vi "Agitator Tags.vi"(11 "AM Module Configs":T1[](array[typedef])) -> (1 "AG Tags":T4, 2 "AM Module Tags Array":T4[](array[typedef]), 3 "All Boolean Tags":string[](array[string]), 4 "All  Numeric Tags":string[](array[string]))   [LabVIEW 2018]
uses:
  Agitator Class/Agitator Module Tag Names.ctl
  Agitator Module Folder/Feed Module/Controls/Agitator Module Config Cluster.ctl
  <vilib>/Utility/miscctls.llb/LVPoint32TypeDef.ctl
  Agitator Module Folder/Feed Module/Controls/Agitator Module Settings Cluster.ctl
  Agitator Module Folder/Agitator Module.lvlib
panel:
  # "Agitator Settings"
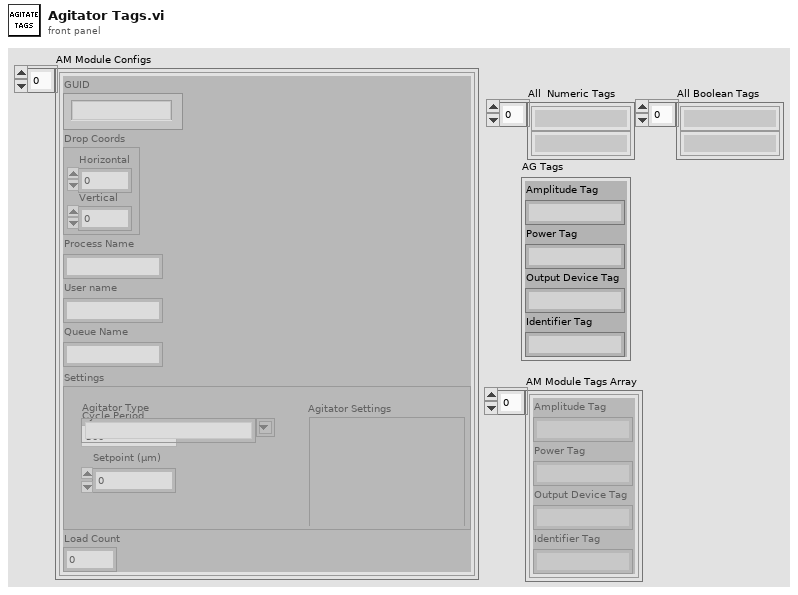
[diagram p1: front panel]
types:
  T1 = typedef "Agitator Module.lvlib/Agitator Module Config Cluster.ctl" = cluster{"GUID":string, "Drop Coords":T2, "Process Name":string, "User name":string, "Queue Name":string, "Settings":T3, "Load Count":i32}
  T2 = typedef "LVPoint32TypeDef.ctl" = cluster{"Horizontal":i32, "Vertical":i32}
  T3 = typedef "Agitator Module.lvlib/Agitator Module Settings Cluster.ctl" = cluster{"Cycle Period":dbl, "Agitator Type":string, "Setpoint (µm)":dbl}
  T4 = typedef "Agitator Module.lvlib/Agitator Module Tag Names.ctl" = cluster{"Amplitude Tag":string, "Power Tag":string, "Output Device Tag":string, "Identifier Tag":string}
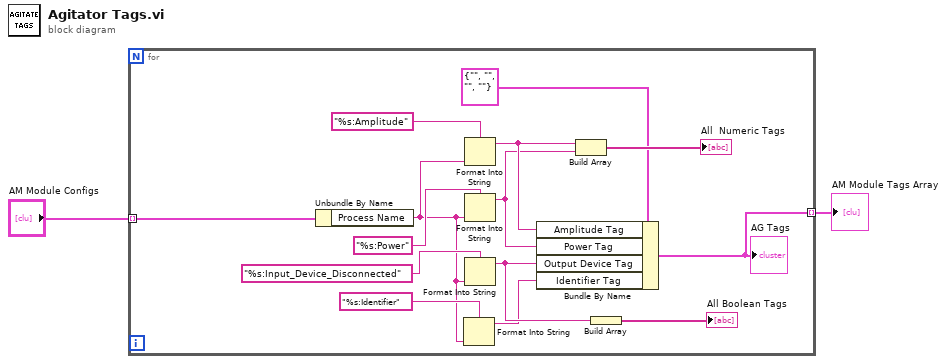
[diagram p0: block diagram]
diagram:
  n1 = for {
    tunnel: [w8] -> w2 mode=indexing
    tunnel: "AM Module Configs" -> [w7] mode=indexing
    n2 = Unbundle By Name(w7) -> ("Process Name"=w4:string)
    n3 = Format Into String(format string="%s:Identifier", w4) -> (resulting string=w3:string)  [unwired: 2 in, 1 out]
    n4 = Format Into String(format string="%s:Amplitude", w4) -> (resulting string=w13:string)  [unwired: 2 in, 1 out]
    n5 = Format Into String(format string="%s:Power", w4) -> (resulting string=w9:string)  [unwired: 2 in, 1 out]
    n6 = Format Into String(format string="%s:Input_Device_Disconnected", w4) -> (resulting string=w11:string)  [unwired: 2 in, 1 out]
    n7 = Bundle By Name(cluster=T4 {"Amplitude Tag"="", "Power Tag"="", "Output Device Tag"="", "Identifier Tag"=""} ("AG Tags"), "Amplitude Tag"=w13, "Power Tag"=w9, "Output Device Tag"=w11, "Identifier Tag"=w3) -> (w8:T4)
    "AG Tags" <- w8
    n8 = Build Array(w13, w9) -> (→"All  Numeric Tags":string[])
    n9 = Build Array(w11) -> (→"All Boolean Tags":string[])
  }
  "AM Module Tags Array" <- w2
